vi "Initialize Datalogger.vi"(8 "error in (no error)":errorcluster, 10 "Base File Path":path, 11 "MWWL Verification in":refnum<class "MWWL Verification.lvclass">) -> (0 "error out":errorcluster, 3 "MWWL Verification out":refnum<class "MWWL Verification.lvclass">)   [LabVIEW 2018, in "MWWL Verification.lvlib" / "MWWL Verification.lvclass"]
uses:
  MWWL Verification.lvclass
  C:/Program Files (x86)/National Instruments/LabVIEW 2018/vi.lib/ActorFramework/Actor/Actor.lvclass
  Datalogger Actor/Datalogger Actor.lvclass
  Datalogger Actor/Datalogger Actor Messages/Configure Datalogger Msg/Configure Datalogger Msg.lvclass/Configure Datalogger Msg.ctl
  <vilib>/ActorFramework/Message Enqueuer/Message Enqueuer.lvclass/Message Enqueuer.ctl
  MWWL Verification.lvclass/MWWL Verification.ctl
  <vilib>/ActorFramework/Message Enqueuer/Enqueue.vi
  Datalogger Actor/Datalogger Actor Messages/Configure Datalogger Msg/Configure Datalogger Msg.lvclass
  C:/Program Files (x86)/National Instruments/LabVIEW 2018/vi.lib/ActorFramework/Message/Message.lvclass
  <vilib>/ActorFramework/Message Priority Queue/Priority Enqueue.vi
  <vilib>/ActorFramework/Actor/Actor.lvclass
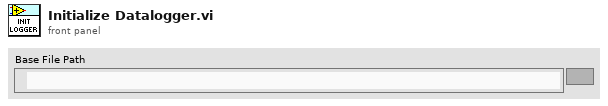
[diagram p1: front panel]
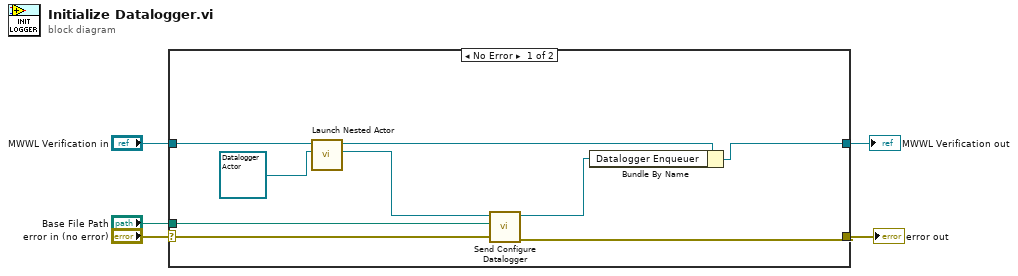
[diagram p0: block diagram]
diagram:
  n1 = case shown="No Error" "error in (no error)" {
    selector: "error in (no error)" -> [w11 w16]
    tunnel: [w7 w16] -> w4
    tunnel: [w12 w15] -> w2
    tunnel: "MWWL Verification in" -> [w13 w15]
    tunnel: "Base File Path" -> [w8 _]
    frame No Error {
      n2 = call <vilib>:"Launch Nested Actor.vi"("Nested Actor"=refnum<class "Datalogger Actor.lvclass"> refnum ("Datalogger Actor.lvlib:Datalogger Actor"), "Caller Actor in"=w13) -> ("Nested Actor's Enqueuer"=w9:refnum<class "Message Enqueuer.lvclass">, "Caller Actor out"=w10:refnum<class "MWWL Verification.lvclass">)  [unwired: 7 in, 1 out]
      n3 = call "Send Configure Datalogger.vi"("error in (no error)"=w11, "Base File Path"=w8, "Message Enqueuer in"=w9) -> ("error out"=w7:errorcluster, "Message Enqueuer out"=w6:refnum<class "Message Enqueuer.lvclass">)  [unwired: 7 in]
      n4 = Bundle By Name(cluster=w10, "Datalogger Enqueuer"=w6) -> (w12:refnum<class "MWWL Verification.lvclass">)
    }
    frame Error {
    }
  }
  "error out" <- w4
  "MWWL Verification out" <- w2
